vi "Read.vi"(8 "error in (no error)":errorcluster, 11 "Websocket Client Handler in":refnum<class "Websocket Client Handler.lvclass">) -> (0 "error out":errorcluster, 3 "Websocket Client Handler out":refnum<class "Websocket Client Handler.lvclass">)   [LabVIEW 2016, in "Stream Mediator.lvlib" / "Websocket Client Handler.lvclass"]
doc: "--\nCopyright © 2017 Composed SystemsI All rights reserved.\n\nAuthor: Jon McBee <jon.mcbee@composed.io>\n\nThis library is provided \"AS IS\" ,WITHOUT WARRANTIES OR\nCONDITIONS OF ANY KIND, either express or implied.\n\nComposed Systems -- composed.io\n\nStream 0.0.1.1\nJon McBee - Composed Systems\nCopyright (c) 2017, Composed Systems"
uses:
  <userlib>/Composed Systems/Stream/Mediator/Classes/Websocket Client Handler Actor/Websocket Client Handler/Websocket Client Handler.lvclass
  C:/Program Files (x86)/National Instruments/LabVIEW 2016/user.lib/Composed Systems/Stream/Mediator/Classes/Mediated Asynchronous Actor/Mediated Asynchronous Actor.lvclass
  <userlib>/Composed Systems/Stream/Mediator/Classes/Websocket Client Handler Actor/Websocket Client Handler Msgs/Read Msg/Read Msg.lvclass
  <userlib>/Composed Systems/Stream/Mediator/Classes/Mediated Asynchronous Actor/Mediated Asynchronous Actor.lvclass
  <userlib>/Composed Systems/Stream/Mediator/Classes/Message Command Stop/Stop Msg.lvclass
  <userlib>/Composed Systems/Stream/Mediator/Classes/Message Transport Queue/Message Transport Queue.lvclass
  C:/Program Files (x86)/National Instruments/LabVIEW 2016/user.lib/Composed Systems/Stream/Mediator/Classes/Message Transport Interface/Message Transport Interface.lvclass
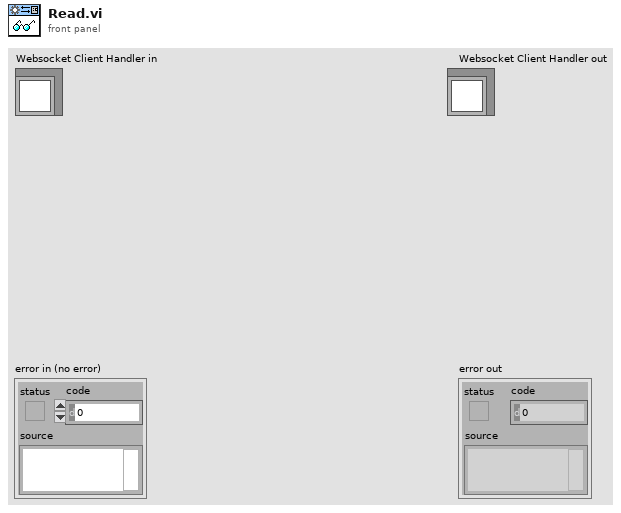
[diagram p1: front panel]
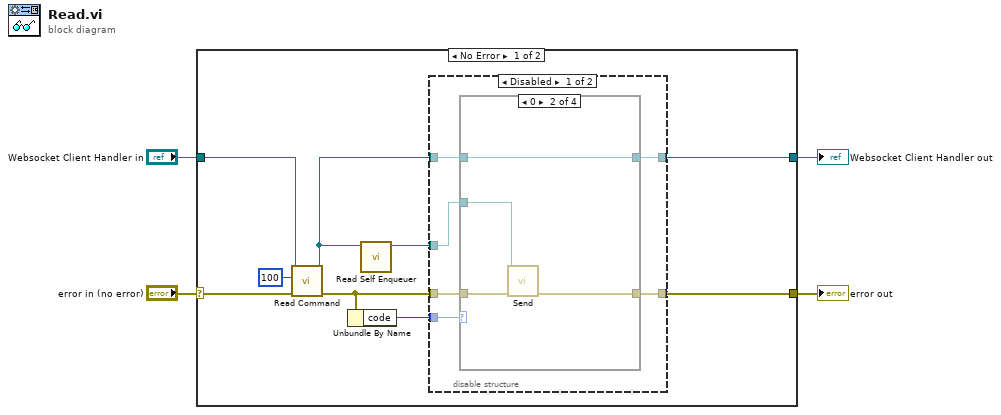
[diagram p0: block diagram]
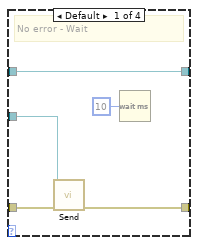
[diagram p2: hidden frame]
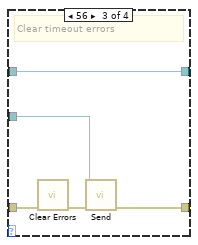
[diagram p3: hidden frame]
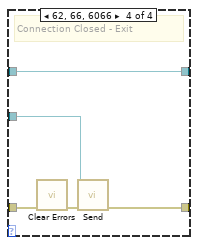
[diagram p4: hidden frame]
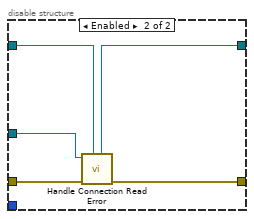
[diagram p5: hidden frame]
diagram:
  n1 = case shown="No Error" "error in (no error)" {
    selector: "error in (no error)" -> [w13 w45]
    tunnel: [w8 w45] -> w3
    tunnel: [w7 w44] -> w1
    tunnel: "Websocket Client Handler in" -> [w12 w44]
    frame No Error {
      n2 = call <userlib>:"Read Command.vi"("error in (no error)"=w13, "timeout ms (5000)"=100, "Websocket Client Handler in"=w12) -> ("error out"=w9:errorcluster, "Websocket Client Handler out"=w6:refnum<class "Websocket Client Handler.lvclass">)  [unwired: 7 in]
      n3 = Unbundle By Name(w9) -> ("code"=w10:i32)
      n4 = call <userlib>:"Read Self Enqueuer.vi"("Mediated Asynchronous Actor in"=w6) -> ("Self Enqueuer"=w5:refnum<class "Message Transport Queue.lvclass">)  [unwired: 10 in]
      n5 = disable-structure shown="Disabled" {
        disable-tunnel: w10 -> [w19 _]
        disable-tunnel: w9 -> [w18 w43]
        disable-tunnel: [w17 w42] -> w8
        disable-tunnel: [w16 w40] -> w7
        disable-tunnel: w6 -> [w15 w41]
        disable-tunnel: w5 -> [w14 w39]
        frame Disabled {
          n6 = case shown="0" w19 {
            tunnel: [w21 w26 w30 w34] -> w17
            tunnel: w18 -> [w22 w27 w33 w38]
            tunnel: [w23 w28 w32 w37] -> w16
            tunnel: w15 -> [w23 w28 w32 w37]
            tunnel: w14 -> [w20 w25 w29 w36]
            frame Default {
              # "No error - Wait"
              n7 = call <userlib>:"Send.vi"("error in (no error)"=w22, "Message Transport Queue"=w20) -> ("error out"=w21:errorcluster)  [unwired: 9 in]
              n8 = Wait (ms)(milliseconds to wait=u32 10) -> ()  [unwired: 1 out]
            }
            frame 0 {
              n9 = call <userlib>:"Send.vi"("error in (no error)"=w27, "Message Transport Queue"=w25) -> ("error out"=w26:errorcluster)  [unwired: 9 in]
            }
            frame 56 {
              # "Clear timeout errors"
              n10 = call <vilib>:"Clear Errors.vi"("error in (no error)"=w33) -> ("error out"=w31:errorcluster)  [unwired: 5 in, 1 out]
              n11 = call <userlib>:"Send.vi"("error in (no error)"=w31, "Message Transport Queue"=w29) -> ("error out"=w30:errorcluster)  [unwired: 9 in]
            }
            frame 62, 66, 6066 {
              # "Connection Closed - Exit"
              n12 = call <vilib>:"Clear Errors.vi"("error in (no error)"=w38) -> ("error out"=w35:errorcluster)  [unwired: 5 in, 1 out]
              n13 = call <userlib>:"Send.vi"("error in (no error)"=w35, "Message Transport"=w36) -> ("error out"=w34:errorcluster)  [unwired: 9 in]
            }
          }
        }
        frame Enabled {
          n14 = call-dynamic "Handle Connection Read Error.vi"("Websocket Client Handler in"=w41, "error in (no error)"=w43, "Self Enqueuer"=w39) -> ("error out"=w42:errorcluster, "Websocket Client Handler out"=w40:refnum<class "Websocket Client Handler.lvclass">)  [unwired: 7 in]
        }
      }
    }
    frame Error {
    }
  }
  "error out" <- w3
  "Websocket Client Handler out" <- w1
